vi "Untitled 1.vi"() -> ()   [LabVIEW 2013]
panel:
  out "Waveform Chart":dbl(graph)
  in  "stop":bool
  in  "Dial":dbl(knob)=0.1 min=0.1 max=2.0 step=0.05 scale=0.0..2.0 scale format="%#.2f"
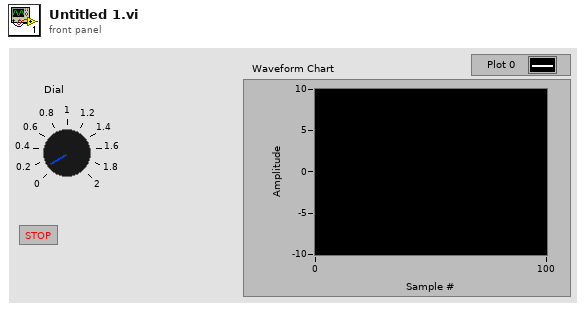
[diagram p1: front panel]
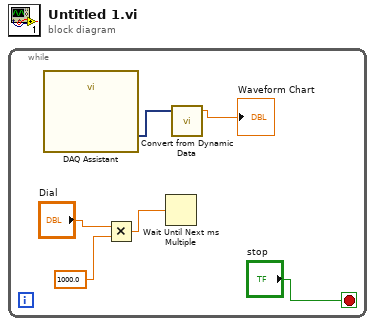
[diagram p0: block diagram]
diagram:
  n1 = while {
    stop <- "stop" stop-if-true
    n2 = call "DAQ Assistant"() -> ("data"=w6:dynamicdata)  [unwired: 17 in, 2 out]
    n3 = Multiply(x="Dial", y=1000.0) -> (x*y=w1:dbl)
    n4 = Wait Until Next ms Multiple(millisecond multiple=w1) -> ()  [unwired: 1 out]
    n5 = call "Convert from Dynamic Data"("Dynamic Data Type"=w6) -> ("Scalar"=→"Waveform Chart":dbl)  [unwired: 3 in]
  }
